vi "GetSetpoint2.vi"(8 "Error In":errorcluster, 11 "Omega CSi32 In":refnum<visa-resource-name>) -> (0 "Error Out":errorcluster, 2 "Setpoint 2 (C)":dbl format="%.1f", 3 "Omega CSi32 Out":refnum<visa-resource-name>)   [LabVIEW 2012, in "Omega-CSi32.lvlib"]
uses:
  Omega-CSi32.lvlib
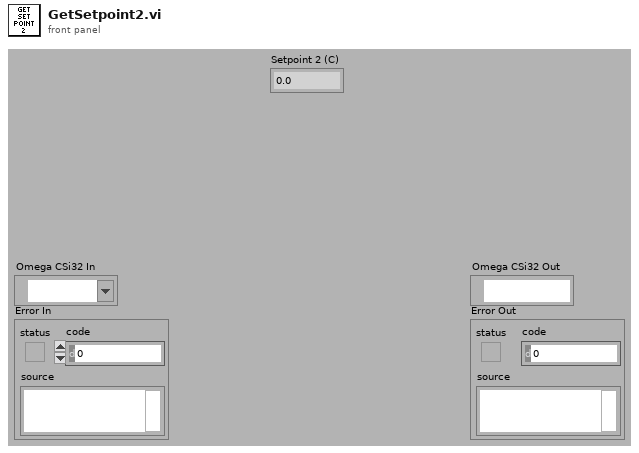
[diagram p1: front panel]
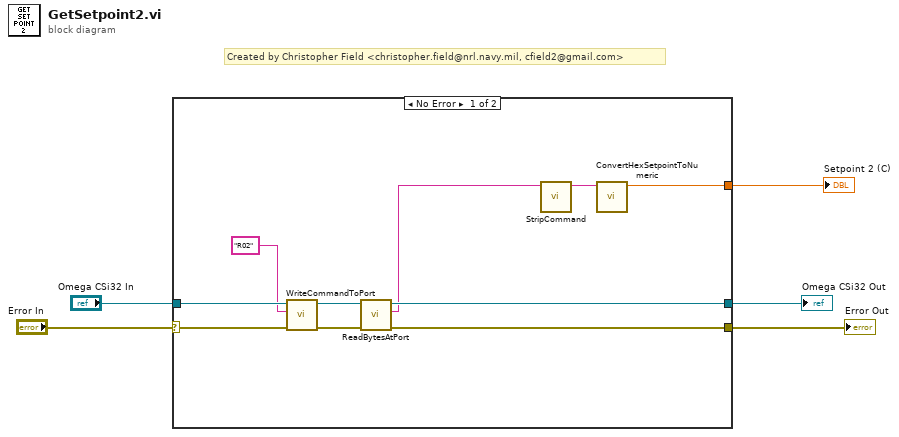
[diagram p0: block diagram]
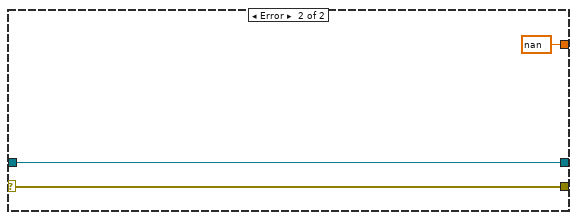
[diagram p2: hidden frame]
diagram:
  # "Created by Christopher Field <christopher.field@nrl.navy.mil, cfield2@gmail.com>"
  n1 = case shown="No Error" "Error In" {
    selector: "Error In" -> [w6 w17]
    tunnel: [w14 nan ("Numeric Setpoint (C)")] -> w5
    tunnel: "Omega CSi32 In" -> [w13 w18]
    tunnel: [w9 w18] -> w3
    tunnel: [w7 w17] -> w2
    frame No Error {
      n2 = call "WriteCommandToPort.vi"("Error In"=w6, "Command"="R02", "CSi32 In"=w13) -> ("Error Out"=w10:errorcluster, "CSi32 Out"=w11:refnum<visa-resource-name>)  [unwired: 7 in]
      n3 = call "ReadBytesAtPort.vi"("Error In"=w10, "CSi32 In"=w11) -> ("Error Out"=w7:errorcluster, "Read Buffer"=w8:string, "CSi32 Out"=w9:refnum<visa-resource-name>)  [unwired: 7 in]
      n4 = call "StripCommand.vi"("Command"=w8) -> ("Stripped Command"=w15:string)  [unwired: 10 in]
      n5 = call "ConvertHexSetpointToNumeric.vi"("Hex Setpoint"=w15) -> ("Numeric Setpoint (C)"=w14:dbl)  [unwired: 10 in]
    }
    frame Error {
    }
  }
  "Omega CSi32 Out" <- w3
  "Error Out" <- w2
  "Setpoint 2 (C)" <- w5
